vi "BRAM_WriteGamePlayfield.vi"(0 "Player IN":u8, 3 "Data":fxp<+,3,3>, 9 "Address":i16) -> (14 "Player OUT":u8)   [LabVIEW 2018]
uses:
  <vilib>/rvi/Memory/Memory_Emulation/nirvimemoryFastEmulation.vi
  <vilib>/rvi/Memory/Memory_Emulation/nirvimemoryEmulation.vi
  <vilib>/rvi/Emulation/niFpgaEmulationIsFPGAContextNoSignature.vi
  <vilib>/rvi/DataTransferAndStorage/Container/Common/niFpgaContainerGetUniqueNameForEmu.vi
  <vilib>/rvi/Emulation/niFpgaProcessEmulError.vi
  <vilib>/rvi/Emulation/niFpgaSctlEmulationGetInTimedLoop.vi
  <vilib>/rvi/errors/nirviReportUnexpectedCaseInternalError (U32).vi
  <vilib>/rvi/DataTransferAndStorage/Container/XNode/niFpgaContainer.xnode
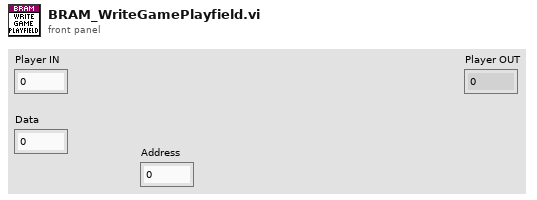
[diagram p1: front panel]
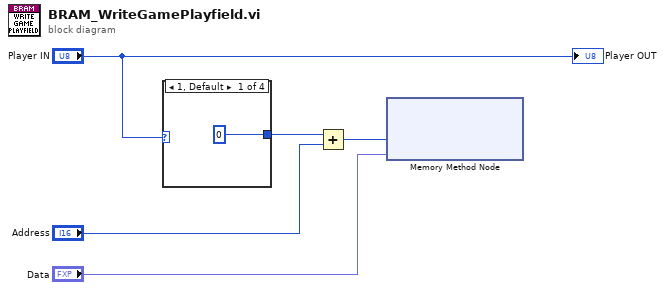
[diagram p0: block diagram]
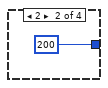
[diagram p2: hidden frame]
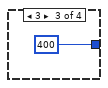
[diagram p3: hidden frame]
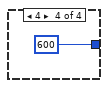
[diagram p4: hidden frame]
diagram:
  n1 = case shown="1, Default" "Player IN" {
    tunnel: [i16 0 ("x") i16 200 ("x") i16 400 ("x") i16 600 ("x")] -> w4
    frame 1, Default {
    }
    frame 2 {
    }
    frame 3 {
    }
    frame 4 {
    }
  }
  n2 = Add(x=w4, y="Address") -> (x+y=w5:i16)
  n3 = xnode ("Memory Method Node")("Address"=w5, "Data"="Data") -> ()  [unwired: 1 in, 1 out]
  "Player OUT" <- "Player IN"
